vi "Tetra_BOUNCE_Setup.vi"() -> (0 "error out":errorcluster, 2 "Status":string="\rSetting up the Power Supplies...\rPower Supplies ON!\rMeasuring DC Power Supply Current(Pre-Boot)\rInitial DC = 0.144814  Amps")   [LabVIEW 2018]
uses:
  <vilib>/Utility/error.llb/DialogType.ctl
  Initialize References/Sequence Globals.vi
  Infrastructure/Test Parameter Globals_1.0.0.vi
  Tetra_Globals.vi
  Initialize References/Station References Global.vi
  Infrastructure/Test Result File Name Global.vi
  <vilib>/Utility/file.llb/Read Delimited Spreadsheet (string).vi
  <vilib>/Utility/file.llb/Write Delimited Spreadsheet (string).vi
panel:
  in  "Controls":T1={"ReadADC"=TRUE, "StartTest"=TRUE, "ResetRFSM"=TRUE, "FtServer"=TRUE, "CalVCO(t)"=TRUE, "Ping(t)"=TRUE, "CmdWindowHide(T)"=FALSE, "OpenNewFt(T)"=TRUE, "UseCmdFile(T)"=FALSE, "#of Retries"=5}
  out "COM PORT":string="COM6"
  out "bad usb connection?(t)":bool
  out "capt_dir":string="#CaptureFileDirectory: 'C:\\RageATE Results\\WAM-C_BOUNCE\\11_28_2022\\WAM-C_BOUNCE_SN_WAM-000102_ 2239_112822-151618_IqCaptureFiles.zip'"
  out "Pmic_FwRev":string
  out "snic":string="#Family: 0x2D\n#Serial: 0x000036092740\r\n"
  out "rev":string="rdiv\r\n0)  sw3p6:   195 mA  3616 mV\r\n1)  sw5p5:    89 mA  5472 mV\r\n2) sw2p8a:   315 mA  2784 mV\r\n3) sw2p8b:   349 mA  2768 mV\r\n4)  sw2p4:  1458 mA  2288 mV\r\n5)  sw1p4:  1047 mA  1304 mV\r\n>"
  out "Tab Control":enum32{"Page 1", "Page 2", "Page 3", "Page 4"}(tab)
  in  "CheckInputClock(T)":bool=TRUE
  in  "Setup Chip (T)":bool=TRUE
  in  "Setup Power Supply (T)":bool=TRUE
  in  "Kill Teraterm":bool=TRUE
  in  "Setup Gantry(t)":bool=TRUE
  out "FPGA_Booted":bool
  out "Ping_Success":bool
  out "Success":bool
  out "AminitOK?(t)":bool=TRUE
  out "Capt_RxIQ_Data(t)":bool=TRUE
  in  "RunFtVco/Ping(t)":bool=TRUE
  out "PyScript(path)":path=path "C:/RageATE/Automated Tests/Tetra WAM/Utilities/VerifySiTime.py"
  out "CMD":string
  out "AppSupportPath":path
  out "IsRuntime?":bool
  out "gui_path":path
  out "ft_path":path
  out "Use PS1-1":bool=TRUE
  out "Temp(t)":bool
  out "Text":refnum<vi>
  out "PS1-1(V)":dbl=18.75
  out "PS1-1(A)":dbl=1.0
  out "Temp Soak(min)":dbl caption="Delay Time (s)"
  out "-dynamic (t)":bool
  out "RunAM_Init(T)":bool
  out "RundynamicMode_Init(T)":bool
  out "PllSuccess?(T)":bool
  out "git log":string="#Gitlog Commit: bb6f7468ffd055d506c281d33be7af8cc293d965   Ver: 1.0.28\n#Gitlog Author: Rick-Rage <74794943+Rick-Rage@users.noreply.github.com>\n#Gitlog Date:   Wed Nov 23 09:45:19 2022 -0500\n#Gitlog ComputerName: HAMPTON"
  out "TEMP":dbl=25.0
  in  "error in (no error)":errorcluster
  # "CLOCK TEST FILES"
types:
  T1 = cluster{"ReadADC":bool, "StartTest":bool, "ResetRFSM":bool, "FtServer":bool, "CalVCO(t)":bool, "Ping(t)":bool, "CmdWindowHide(T)":bool, "OpenNewFt(T)":bool, "UseCmdFile(T)":bool, "#of Retries":i32}
  T2 = typedef "DialogType.ctl" = u16
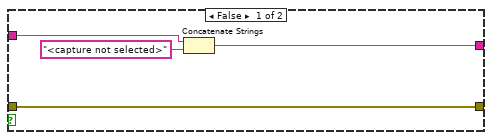
[diagram p3: hidden frame]
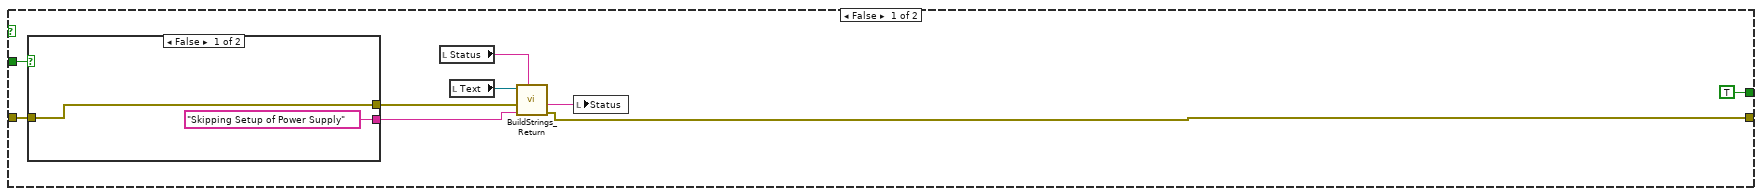
[diagram p5: hidden frame]
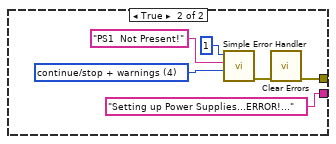
[diagram p6: hidden frame]
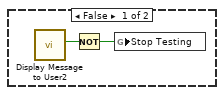
[diagram p8: hidden frame]
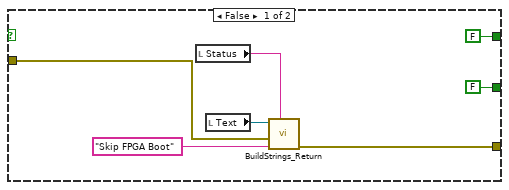
[diagram p10: hidden frame]
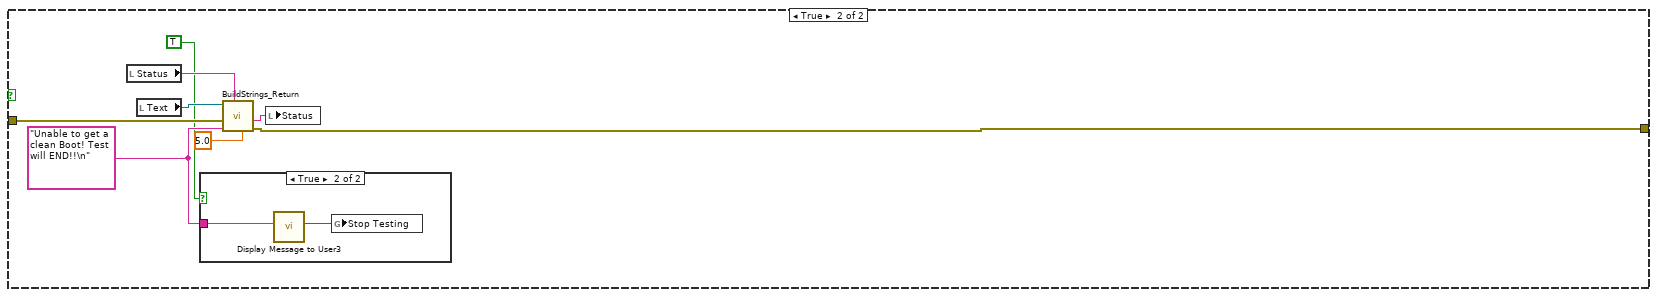
[diagram p11: hidden frame]
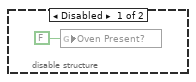
[diagram p13: hidden frame]
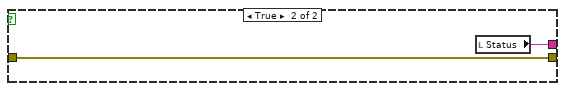
[diagram p14: hidden frame]
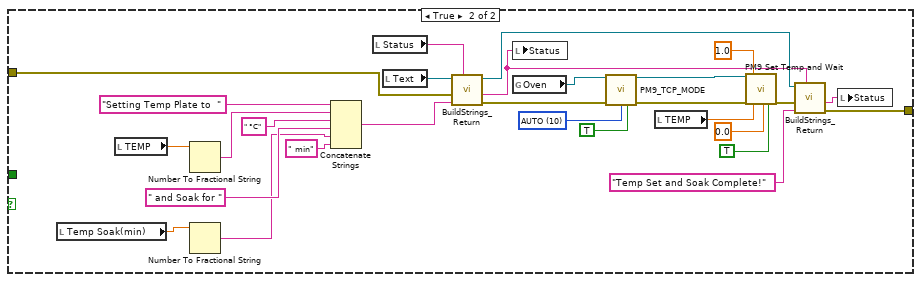
[diagram p15: hidden frame]
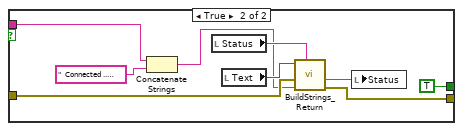
[diagram p17: hidden frame]
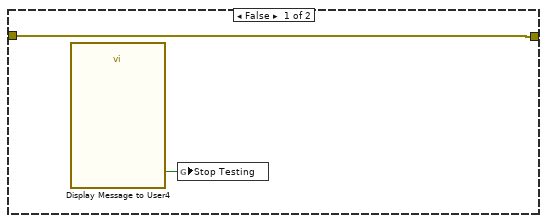
[diagram p19: hidden frame]
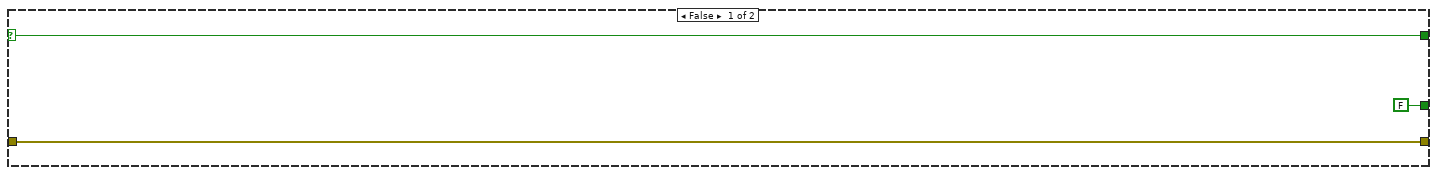
[diagram p20: hidden frame]
diagram:
  n1 = flat-sequence {
    tunnel: [w38] -> w15
    tunnel: w15 -> [w57]
    tunnel: [w56] -> w14
    tunnel: [w55] -> w13
    tunnel: [w53] -> w6
    tunnel: [w71] -> w7
    tunnel: w14 -> [w78]
    tunnel: w13 -> [w77]
    tunnel: w6 -> [w71]
    tunnel: [w81] -> w12
    tunnel: w7 -> [w80]
    tunnel: w12 -> [w103]
    tunnel: [w102] -> w11
    tunnel: [w113] -> w9
    tunnel: w11 -> [w112]
    tunnel: [w111] -> w1
    tunnel: w9 -> [w182]
    tunnel: [w181] -> w4
    tunnel: w1 -> [w180]
    tunnel: [w242] -> w5
    tunnel: w4 -> [w241]
    tunnel: [w293] -> w8
    tunnel: w5 -> [w294]
    tunnel: [w338] -> w3
    tunnel: w8 -> [w337]
    tunnel: w3 -> [w425]
    tunnel: [w424] -> w2
    tunnel: [w473] -> w10
    tunnel: w2 -> [w484]
    frame #0 {
      w16 = FALSE ("FPGA_Booted")
      # "Kill TeraTerm"
      n2 = flat-sequence {
        frame #0 {
          # "Clock Test References"
          n3 = global read "Sequence Globals.vi" "DevSupportPath"() -> (w43:path)
          n4 = global read "Sequence Globals.vi" "AppSupportPath"() -> (w45:path)
          "AppSupportPath" <- w45
          n5 = Strip Path(path=w43) -> (stripped path=w42:path)  [unwired: 1 out]
          n6 = global read "Sequence Globals.vi" "IsRuntime?"() -> (w46:bool)
          "IsRuntime?" <- w46
          n7 = Build Path(base path=w42, name or relative path=path "Utilities/VerifySiTime.py" ("PyScript(path)")) -> (appended path=w40:path)
          n8 = Select(t=w45, s=w46, f=w40) -> (s? t:f=w44:path)
          "PyScript(path)" <- w44
          n9 = local write "PyScript(path)"(w44) -> ()
        }
      }
      n10 = global read "Sequence Globals.vi" "DevSupportPath"() -> (w28:path)
      n11 = global read "Sequence Globals.vi" "DevSupportPath"() -> (w18:path)
      n12 = global read "Sequence Globals.vi" "RageATE_Gitlog"() -> (→"git log":string)
      n13 = local write "AminitOK?(t)"(w16) -> ()
      n14 = global read "Sequence Globals.vi" "AppSupportPath 3"() -> (w23:path)
      n15 = global read "Sequence Globals.vi" "AppSupportPath 3"() -> (w22:path)
      n16 = global read "Sequence Globals.vi" "IsRuntime?"() -> (w24:bool)
      n17 = global read "Sequence Globals.vi" "IsRuntime?"() -> (w21:bool)
      n18 = local write "Setup Gantry(t)"("Setup Gantry(t)") -> ()
      n19 = local write "Setup Chip (T)"("Setup Chip (T)") -> ()
      n20 = Build Path(base path=w28, name or relative path=path "TetraLabGUI" ("PyScript(path)")) -> (appended path=w26:path)
      n21 = Build Path(base path=w18, name or relative path=path "FieldTestApp" ("PyScript(path)")) -> (appended path=w20:path)
      n22 = local write "Setup Power Supply (T)"("Setup Power Supply (T)") -> ()
      n23 = Select(t=w23, s=w24, f=w26) -> (s? t:f=→"gui_path":path)
      n24 = Select(t=w22, s=w21, f=w20) -> (s? t:f=→"ft_path":path)
      n25 = case shown="True" "Kill Teraterm" {
        tunnel: "error in (no error)" -> [w47 w49]
        tunnel: [w47 w48] -> w38
        tunnel: "taskkill /f /im ttermpro.exe" ("command line") -> [_ w51]
        frame False {
        }
        frame True {
          n26 = call <vilib>:"Clear Errors.vi"("error in (no error)"=w49) -> ("error out"=w50:errorcluster)  [unwired: 5 in, 1 out]
          n27 = call <vilib>:"System Exec.vi"("error in (no error)"=w50, "command line"=w51) -> ("error out"=w52:errorcluster)  [unwired: 6 in, 3 out]
          n28 = call "Time Delay2"("error in (no error)"=w52) -> ("error out"=w48:errorcluster)  [unwired: 10 in]
        }
      }
      "Success" <- FALSE ("Success")
      "Status" <- ""
      "Tab Control" <- enum32{"Page 1", "Page 2", "Page 3", "Page 4"}."Page 1" ("Tab Control")
      "RundynamicMode_Init(T)" <- w16
      "RunAM_Init(T)" <- w16
      "-dynamic (t)" <- w16
    }
    frame #1 {
      # "0\t0\tCOMPORT\tname\n1\t0\tPS1-1 V;I\tVolt : Amp\n2\t0\tCycle_Power\tBool\n3\t0\tAverages\tnum\n4\t0\tCreate_iq_File\tbool\n5\t0\tTemp_Soak\tsec\n6\t0\tCMD\tcommand line\n7\t0\tUse_Gantry\tBool"
      n29 = property on="Status" class="Str"(error in=w57) -> (error out=w53:errorcluster, "Text"=→"Text":refnum<vi>)  [unwired: 1 in, 1 out]
      n30 = global read "Test Parameter Globals_1.0.0.vi" "Input Constants Out"() -> (w56:string[])
      n31 = global read "Test Parameter Globals_1.0.0.vi" "Test Parameters"() -> (w55:string[][])
    }
    frame #2 {
      w64 = 0 ("index (row)")
      n32 = Index Array(array=w78) -> (element #1=w63:string, element #2=w58:string, element #5=w62:string, element #6=w61:string, element #7=→"CMD":string, element #8=w59:string)  [unwired: 8 in, 2 out]
      n33 = Index Array(array=w77, index (row)=w64, index (col)=w64) -> (element=w65:string)
      n34 = global read "Tetra_Globals.vi" "comport"() -> (w67:refnum<visa-resource-name>)
      n35 = Empty String/Path?(string/path=w63) -> (empty?=w69:bool)
      n36 = call "TempControlWithBool.vi"("INPUT"=w65) -> ("out"=→"TEMP":dbl, "Valid(t)"=w75:bool)  [unwired: 6 in, 1 out]
      "Temp(t)" <- w75
      n37 = call "StringToNumberControlWithBool(x2).vi"("string"=w58) -> ("Num(2)"=→"PS1-1(A)":dbl, "Num"=→"PS1-1(V)":dbl, "NOT_0?"=→"Use PS1-1":bool)  [unwired: 4 in, 4 out]
      n38 = call "StringToNumberControlWithBool.vi"("String In"=w62) -> ("NOT = 0"=→"Capt_RxIQ_Data(t)":bool)  [unwired: 7 in, 1 out]
      n39 = call "StringToNumberControlWithBool.vi"("String In"=w61) -> ("Number Out"=→"Temp Soak(min)":dbl)  [unwired: 7 in, 1 out]
      n40 = call "StringToNumberControlWithBool.vi"("String In"=w59) -> ("NOT = 0"=w66:bool)  [unwired: 7 in, 1 out]
      n41 = Select(t=w67, s=w69, f=w58) -> (s? t:f=→"COM PORT":refnum<visa-resource-name>)
      n42 = global write "Station References Global.vi" "Oven Present?"(w75) -> ()
      n43 = local write "Setup Gantry(t)"(w66) -> ()
    }
    frame #3 {
      n44 = flat-sequence {
        tunnel: w80 -> [w86]
        tunnel: [w85] -> w81
        frame #0 {
          n45 = local read "Capt_RxIQ_Data(t)"() -> (w82:bool)
          n46 = case shown="True" w82 {
            tunnel: [w87 w93] -> w84
            tunnel: w86 -> [w90 w97]
            tunnel: [w90 w96] -> w85
            tunnel: "#CaptureFileDirectory: " ("string") -> [w89 w95]
            frame False {
              n47 = Concatenate Strings(w89, "<capture not selected>" ("string")) -> (w87:string)
            }
            frame True {
              w94 = "'" ("string")
              # "For Header"
              n48 = global read "Test Result File Name Global.vi" "Test Results File Name"() -> (w101:path)
              n49 = Path To String(path=w101) -> (string=w100:string)
              n50 = Search and Replace String(input string=w100, search string=".csv", replace string="_Iq.csv" ("name or relative path"), error in=w97) -> (result string=w91:string, error out=w96:errorcluster)  [unwired: 4 in, 2 out]
              n51 = String To Path(string=w91) -> (path=w92:path)
              n52 = Concatenate Strings(w95, w94, w91, w94) -> (w93:string)
              n53 = global write "Tetra_Globals.vi" "TraceFilePath"(w92) -> ()
            }
          }
          "capt_dir" <- w84
        }
      }
    }
    frame #4 {
      n54 = global read "Station References Global.vi" "RF Switch Present?"() -> (w104:bool)
      n55 = case shown="True" w104 {
        tunnel: w103 -> [w105 w109]
        tunnel: [w105 w108] -> w102
        frame False {
        }
        frame True {
          n56 = global read "Station References Global.vi" "RF Switch"() -> (w110:refnum<visa-resource-name>)
          n57 = call "RfSwitch_WAM_ATE.vi"("VISA_IN"=w110, "error in"=w109, "Source"=enum16{"RFSM", "PNA"}."RFSM", "T/R"=enum16{"TX", "RX"}."RX") -> ("error out"=w108:errorcluster)  [unwired: 10 in, 1 out]
        }
      }
    }
    frame #5 {
      n58 = local read "Setup Power Supply (T)"() -> (w114:bool)
      n59 = global read "Station References Global.vi" "PS1 Present?"() -> (w116:bool)
      n60 = And(x=w116, y=w114) -> (x .and. y?=w115:bool)
      n61 = case shown="True" w115 {
        tunnel: [w119 w140] -> w113
        tunnel: w114 -> [w125 _]
        tunnel: w112 -> [w118 w139]
        tunnel: [TRUE w134] -> w111
        frame False {
          n62 = case shown="False" w125 {
            tunnel: [w126 w129] -> w120
            tunnel: ["Skipping Setup of Power Supply" "Setting up Power Supplies...ERROR!..."] -> w121
            tunnel: w118 -> [w126 _]
            frame False {
            }
            frame True {
              w131 = T2 4 items=["no dialog", "OK message", "continue or stop message", "OK message + warnings", "continue/stop + warnings"] ("type of dialog (OK msg:1)")
              n63 = call <vilib>:"Simple Error Handler.vi"("error code (no error:0)"=1, "error source (\" \")"="PS1  Not Present!" ("error source (\" \")"), "type of dialog (OK msg:1)"=w131) -> ("error out"=w130:errorcluster)  [unwired: 2 in, 4 out]
              n64 = call <vilib>:"Clear Errors.vi"("error in (no error)"=w130) -> ("error out"=w129:errorcluster)  [unwired: 5 in, 1 out]
            }
          }
          n65 = local read "Status"() -> (w122:string)
          n66 = local read "Text"() -> (w124:refnum<vi>)
          n67 = call "BuildStrings_Return.vi"("Input String"=w122, "New String"=w121, "error in (no error)"=w120, "reference"=w124) -> ("error out"=w119:errorcluster, "concatenated string"=w123:string)  [unwired: 5 in, 1 out]
          n68 = local write "Status"(w123) -> ()
        }
        frame True {
          n69 = control-ref of="Text"() -> ()  [unwired: 1 out]
          n70 = for {
            N: 2 -> [w145]
            shift-right: [w150] -> w140
            shift-left: w139 -> [w146]
            tunnel: [w142] -> w137
            tunnel: [w141] -> w136
            i -> [w144]
            stop <- w141 stop-if-true
            w148 = TRUE ("Open Ser(t)")
            n71 = Increment(x=w144) -> (x+1=w143:i32)
            n72 = Equal?(x=w145, y=w143) -> (x = y?=w142:bool)
            n73 = local read "Status"() -> (w159:string)
            n74 = local read "Text"() -> (w158:refnum<vi>)
            n75 = call "BuildStrings_Return.vi"("Input String"=w159, "New String"="Setting up the Power Supplies...", "error in (no error)"=w146, "reference"=w158) -> ("error out"=w160:errorcluster, "concatenated string"=w157:string)  [unwired: 5 in, 1 out]
            n76 = local write "Status"(w157) -> ()
            n77 = stacked-sequence {
              tunnel: w160 -> [w179]
              tunnel: [w178] -> w154
              tunnel: [w165] -> _
              tunnel: [w164] -> _
              frame #0 {
                w167 = "PS1" ("SEL_PS")
                # "Conf I/V lim"
                n78 = local read "Text"() -> (w170:refnum<vi>)
                n79 = local read "PS1-1(A)"() -> (w176:dbl)
                n80 = local read "PS1-1(V)"() -> (w175:dbl)
                n81 = property class="Txt"(reference=w170, error in=w179, "Scroll Position"=i16 -1) -> (error out=w168:errorcluster)  [unwired: 1 out]
                n82 = global read "Station References Global.vi" "PS1"() -> (w177:refnum<visa-resource-name>)
                n83 = Build Array(w176, 1.0 ("element")) -> (w165:dbl[])
                n84 = Build Array(w175, 5.0 ("element")) -> (w164:dbl[])
                n85 = call "PS_SETUP_V-I-EN.vi"("VISA resource name"=w177, "SEL_PS"=w167, "error in (no error)"=w168, "Use Channel"=bool[] [FALSE, FALSE, FALSE, FALSE], "Current Lim"=w165, "Voltage Set"=w164) -> ("VISA resource name out"=w171:refnum<visa-resource-name>, "error out"=w173:errorcluster)  [unwired: 8 in]
                n86 = call "Time Delay5"("error in (no error)"=w173) -> ("error out"=w166:errorcluster)  [unwired: 10 in]
                n87 = call "PS_SETUP_V-I-EN.vi"("VISA resource name"=w171, "SEL_PS"=w167, "error in (no error)"=w166, "Use Channel"=bool[] [TRUE, FALSE, FALSE, FALSE], "Current Lim"=w165, "Voltage Set"=w164) -> ("error out"=w178:errorcluster)  [unwired: 8 in, 1 out]
              }
            }
            n88 = local read "Text"() -> (w156:refnum<vi>)
            n89 = local read "COM PORT"() -> (w149:string)
            n90 = call "BuildStrings_Return.vi"("seconds to wait"=5.0, "Input String"=w157, "New String"="Power Supplies ON!", "error in (no error)"=w154, "reference"=w156) -> ("error out"=w151:errorcluster, "concatenated string"=w153:string)  [unwired: 4 in, 1 out]
            n91 = local write "Status"(w153) -> ()
            n92 = call "Tetra Serial.vi"("COMPORT"=w149, "ClearErrorIn(t)"=TRUE, "error in (no error)"=w151, "Open Ser(t)"=w148, "Close Ser(t)"=w148) -> ("Success"=w141:bool, "error out"=w150:errorcluster)  [unwired: 6 in, 3 out]
          }
          n93 = Not(x=w136) -> (.not. x?=w135:bool)
          n94 = And(x=w137, y=w135) -> (x .and. y?=w134:bool)
          "bad usb connection?(t)" <- w134
        }
      }
    }
    frame #6 {
      n95 = case shown="False" w180 {
        tunnel: w182 -> [w184 w234]
        tunnel: [w183 w230] -> w181
        frame False {
          n96 = flat-sequence {
            tunnel: w184 -> [w192]
            tunnel: [w187] -> w183
            frame #0 {
              n97 = local read "Setup Chip (T)"() -> (w193:bool)
              n98 = case shown="True" w193 {
                selector: w193 -> [_ w217]
                tunnel: [FALSE ("Success") w229] -> w188
                tunnel: [w210 w216] -> w191
                tunnel: w192 -> [w211 w220]
                tunnel: [FALSE w217] -> w189
                frame False {
                  n99 = local read "Status"() -> (w212:string)
                  n100 = local read "Text"() -> (w213:refnum<vi>)
                  n101 = call "BuildStrings_Return.vi"("Input String"=w212, "New String"="Skip FPGA Boot", "error in (no error)"=w211, "reference"=w213) -> ("error out"=w210:errorcluster)  [unwired: 5 in, 2 out]
                }
                frame True {
                  n102 = local read "Status"() -> (w224:string)
                  n103 = local read "Text"() -> (w223:refnum<vi>)
                  n104 = call "BuildStrings_Return.vi"("seconds to wait"=0.0, "Input String"=w224, "New String"="Booting up FPGA...\nTakes up to 10sec..." ("Delay text ..."), "error in (no error)"=w220, "reference"=w223) -> ("error out"=w219:errorcluster, "concatenated string"=w218:string)  [unwired: 4 in, 1 out]
                  n105 = local read "COM PORT"() -> (w226:string)
                  n106 = local write "Status"(w218) -> ()
                  n107 = call "Tetra Serial.vi"("COMPORT"=w226, "error in (no error)"=w219, "Command"="", "Open Ser(t)"=TRUE, "Close Ser(t)"=FALSE) -> ("Success"=w229:bool, "error out"=w216:errorcluster)  [unwired: 6 in, 3 out]
                }
              }
              n108 = And(x=w188, y=w189) -> (x .and. y?=w190:bool)
              n109 = local write "FPGA_Booted"(w188) -> ()
              n110 = case shown="True" w190 {
                tunnel: w191 -> [w202 w207]
                tunnel: [w202 w203] -> w186
                frame False {
                }
                frame True {
                  n111 = local read "Status"() -> (w206:string)
                  n112 = local read "Text"() -> (w208:refnum<vi>)
                  n113 = call "BuildStrings_Return.vi"("Input String"=w206, "New String"="FPGA Success!!", "error in (no error)"=w207, "reference"=w208) -> ("error out"=w203:errorcluster, "concatenated string"=w204:string)  [unwired: 5 in, 1 out]
                  n114 = local write "Status"(w204) -> ()
                }
              }
              n115 = local read "CheckInputClock(T)"() -> (w185:bool)
              n116 = case shown="True" w185 {
                tunnel: [w194 w199] -> w187
                tunnel: w186 -> [w194 w198]
                frame False {
                }
                frame True {
                  w195 = u16 0 items=["EXT CLK", "INT CLK"] ("CLK_USAGE")
                  n117 = local read "COM PORT"() -> (w196:string)
                  n118 = call "InputClk_Status.vi"("COMPORT"=w196, "error in (no error)"=w198, "CLK_USAGE"=w195) -> ("PllSuccess?(T)"=w197:bool, "error out"=w199:errorcluster)  [unwired: 11 in]
                  "PllSuccess?(T)" <- w197
                  n119 = case shown="True" w197 {
                    frame False {
                      n120 = call "Display Message to User2"() -> ("OK"=w201:bool)  [unwired: 10 in, 1 out]
                      n121 = Not(x=w201) -> (.not. x?=w200:bool)
                      n122 = global write "Sequence Globals.vi" "Stop Testing"(w200) -> ()
                    }
                    frame True {
                    }
                  }
                }
              }
            }
          }
        }
        frame True {
          w232 = "Unable to get a clean Boot! Test will END!!\n" ("New String")
          n123 = local read "Status"() -> (w233:string)
          n124 = local read "Text"() -> (w235:refnum<vi>)
          n125 = case shown="True" TRUE {
            tunnel: w232 -> [_ w239]
            frame False {
            }
            frame True {
              n126 = call "Display Message to User3"("Message"=w239) -> ("OK"=w238:bool)  [unwired: 9 in, 1 out]
              n127 = global write "Sequence Globals.vi" "Stop Testing"(w238) -> ()
            }
          }
          n128 = call "BuildStrings_Return.vi"("seconds to wait"=5.0, "Input String"=w233, "New String"=w232, "error in (no error)"=w234, "reference"=w235) -> ("error out"=w230:errorcluster, "concatenated string"=w236:string)  [unwired: 4 in, 1 out]
          n129 = local write "Status"(w236) -> ()
        }
      }
    }
    frame #7 {
      n130 = global read "Sequence Globals.vi" "Stop Testing"() -> (w240:bool)
      n131 = case shown="False" w240 {
        tunnel: [w244 w291] -> w242
        tunnel: w241 -> [w243 w291]
        frame False {
          n132 = global read "Station References Global.vi" "Oven Present?"() -> (w245:bool)
          n133 = local read "Temp(t)"() -> (w246:bool)
          n134 = And(x=w246, y=w245) -> (x .and. y?=w247:bool)
          n135 = case shown="False" w247 {
            tunnel: w246 -> [w253 _]
            tunnel: [w251 w273] -> w244
            tunnel: w243 -> [w248 w286]
            frame False {
              n136 = disable-structure shown="Enabled" {
                frame Disabled {
                  n137 = global write "Station References Global.vi" "Oven Present?"(FALSE ("Oven Present?")) -> ()
                }
                frame Enabled {
                }
              }
              n138 = call "Display Message to User"("error in (no error)"=w248, "Enable"=w253) -> ("error out"=w250:errorcluster, "Cancel"=w252:bool)  [unwired: 8 in]
              n139 = Stop(stop? (T)=w252) -> ()
              n140 = case shown="False" w252 {
                tunnel: [w259 w261] -> w249
                tunnel: [w258 w262] -> w251
                tunnel: w250 -> [w257 w262]
                frame False {
                  n141 = local read "Status"() -> (w255:string)
                  n142 = local read "Text"() -> (w256:refnum<vi>)
                  n143 = call "BuildStrings_Return.vi"("Input String"=w255, "New String"="Skipping Setting Up Temperature...", "error in (no error)"=w257, "reference"=w256) -> ("error out"=w258:errorcluster, "concatenated string"=w259:string)  [unwired: 5 in, 1 out]
                }
                frame True {
                  n144 = local read "Status"() -> (w261:string)
                }
              }
              n145 = local write "Status"(w249) -> ()
            }
            frame True {
              w281 = u16 10 items=["READ ONLY"=0, "AUTO"=10, "OFF"=62, "MAN"=54] ("MODE")
              n146 = local read "Temp Soak(min)"() -> (w269:dbl)
              n147 = local read "TEMP"() -> (w276:dbl)
              n148 = Number To Fractional String(number=w276) -> (F-format string=w275:string)  [unwired: 3 in]
              n149 = Number To Fractional String(number=w269) -> (F-format string=w267:string)  [unwired: 3 in]
              n150 = Concatenate Strings("Setting Temp Plate to  ", w275, " °C" ("string"), " and Soak for " ("string"), w267, " min" ("string")) -> (w277:string)
              n151 = local read "Status"() -> (w278:string)
              n152 = local read "Text"() -> (w279:refnum<vi>)
              n153 = call "BuildStrings_Return.vi"("Input String"=w278, "New String"=w277, "error in (no error)"=w286, "reference"=w279) -> ("error out"=w283:errorcluster, "concatenated string"=w264:string, "reference out"=w271:refnum<vi>)  [unwired: 5 in]
              n154 = local write "Status"(w264) -> ()
              n155 = global read "Station References Global.vi" "Oven"() -> (w284:refnum<visa-resource-name>)
              n156 = call "PM9_TCP_MODE.vi"("VISA"=w284, "error in (no error)"=w283, "MODE"=w281, "Close tcp(t)"=TRUE) -> ("visa out"=w280:refnum<visa-resource-name>, "error out"=w285:errorcluster)  [unwired: 8 in, 2 out]
              n157 = local read "TEMP"() -> (w289:dbl)
              n158 = call "PM9 Set Temp and Wait.vi"("VISA"=w280, "Error In"=w285, "Accuracy +/-"=1.0, "Set Point"=w289, "Min (-1 for cont.)"=0.0, "close session(t)"=TRUE) -> ("error out"=w272:errorcluster)  [unwired: 10 in, 3 out]
              n159 = call "BuildStrings_Return.vi"("Input String"=w264, "New String"="Temp Set and Soak Complete!", "error in (no error)"=w272, "reference"=w271) -> ("error out"=w273:errorcluster, "concatenated string"=w270:string)  [unwired: 5 in, 1 out]
              n160 = local write "Status"(w270) -> ()
            }
          }
        }
        frame True {
        }
      }
    }
    frame #8 {
      n161 = global read "Sequence Globals.vi" "Stop Testing"() -> (w292:bool)
      n162 = case shown="False" w292 {
        tunnel: w294 -> [w300 w335]
        tunnel: [w299 w335] -> w293
        frame False {
          n163 = for {
            N: 2 -> [_]
            shift-right: [w306] -> w299
            shift-left: w300 -> [w310]
            tunnel: [w303] -> w298
            stop <- w303 stop-if-true
            n164 = local read "Status"() -> (w311:string)
            n165 = local read "Text"() -> (w313:refnum<vi>)
            n166 = call "BuildStrings_Return.vi"("seconds to wait"=1.0, "Input String"=w311, "New String"="Checking IP Address: 169.254.70.191, for Fast RxData", "error in (no error)"=w310, "reference"=w313) -> ("error out"=w307:errorcluster, "concatenated string"=w309:string)  [unwired: 4 in, 1 out]
            n167 = local write "Status"(w309) -> ()
            n168 = call "PingCmdLine.vi"("error in (no error)"=w307, "IP Address"="169.254.70.191" ("IP_ADDR")) -> ("error out"=w308:errorcluster, "Match?(t)"=w301:bool, "Ip_out"=w302:string)  [unwired: 7 in]
            n169 = case shown="False" w301 {
              tunnel: w308 -> [w319 w331]
              tunnel: [w317 w330] -> w306
              tunnel: [w316 TRUE] -> w303
              tunnel: w302 -> [w314 w326]
              frame False {
                n170 = Concatenate Strings("Failed to Connect to " ("New String"), w314, "Check Address and Connections" ("string")) -> (w322:string)
                n171 = local read "Status"() -> (w324:string)
                n172 = local read "Text"() -> (w323:refnum<vi>)
                n173 = call "BuildStrings_Return.vi"("Input String"=w324, "New String"=w322, "error in (no error)"=w319, "reference"=w323) -> ("error out"=w318:errorcluster, "concatenated string"=w325:string)  [unwired: 5 in, 1 out]
                n174 = local write "Status"(w325) -> ()
                n175 = call "Prompt User for Input2"("Enable"=TRUE, "error in (no error)"=w318) -> ("OK"=w316:bool, "error out"=w317:errorcluster)  [unwired: 16 in]
              }
              frame True {
                n176 = Concatenate Strings(w326, "  Connected ..Success!!" ("New String")) -> (w329:string)
                n177 = local read "Status"() -> (w333:string)
                n178 = local read "Text"() -> (w332:refnum<vi>)
                n179 = call "BuildStrings_Return.vi"("Input String"=w333, "New String"=w329, "error in (no error)"=w331, "reference"=w332) -> ("error out"=w330:errorcluster, "concatenated string"=w334:string)  [unwired: 5 in, 1 out]
                n180 = local write "Status"(w334) -> ()
              }
            }
            n181 = local write "Ping_Success"(w303) -> ()
          }
          n182 = local read "FPGA_Booted"() -> (w296:bool)
          n183 = And(x=w296, y=w298) -> (x .and. y?=w297:bool)
          n184 = local write "Success"(w297) -> ()
        }
        frame True {
        }
      }
    }
    frame #9 {
      n185 = global read "Sequence Globals.vi" "Stop Testing"() -> (w336:bool)
      n186 = case shown="False" w336 {
        tunnel: [w347 w422] -> w338
        tunnel: w337 -> [w340 w422]
        frame False {
          n187 = local read "Setup Chip (T)"() -> (w342:bool)
          n188 = local read "Success"() -> (w341:bool)
          n189 = And(x=w342, y=w341) -> (x .and. y?=w343:bool)
          n190 = case shown="True" w343 {
            selector: w343 -> [w374 w403]
            tunnel: w340 -> [w375 w382]
            tunnel: [w375 w378] -> w345
            tunnel: [w374 w403] -> w346
            tunnel: [FALSE ("OK?(t)") w376] -> w339
            frame False {
            }
            frame True {
              n191 = local read "CMD"() -> (w391:string)
              n192 = Empty String/Path?(string/path=w391) -> (empty?=w392:bool)
              n193 = case shown="False" w392 {
                tunnel: [w419 ""] -> w381
                tunnel: w391 -> [w418 _]
                frame False {
                  n194 = Concatenate Strings(";" ("string"), w418) -> (w419:string)
                }
                frame True {
                }
              }
              n195 = local read "COM PORT"() -> (w383:string)
              n196 = call "SerRW-Array.vi"("COMPORT"=w383, "error in (no error)"=w382, "Command ( ; seperation)"=w381, "Open Serial"=FALSE ("Open/Close Serial")) -> ("comport"=w395:refnum<visa-resource-name>, "error out"=w394:errorcluster)  [unwired: 5 in, 5 out]
              n197 = global read "Tetra_Globals.vi" "BarCodeESN"() -> (w384:string)
              n198 = call "Tetra_Rev.vi"("COMPORT"=w395, "error in (no error)"=w394) -> ("rev"=→"rev":string, "comport"=w401:refnum<visa-resource-name>, "error out"=w400:errorcluster)  [unwired: 9 in, 2 out]
              n199 = call "Tetra_ReadESN.vi"("COMPORT"=w401, "BC_Esn"=w384, "error in (no error)"=w400) -> ("read"=→"snic":string, "comport"=w387:refnum<visa-resource-name>, "esn"=w398:string, "error out"=w389:errorcluster)  [unwired: 8 in, 1 out]
              n200 = global write "Tetra_Globals.vi" "ESN"(w398) -> ()
              n201 = call "ESNLookup.vi"("ESN"=w398, "error in"=w389) -> ("error out"=w388:errorcluster)  [unwired: 7 in, 2 out]
              n202 = call "UCD_Device-Info.vi"("COMPORT"=w387, "error in (no error)"=w388) -> ("Pmic_FwRev"=→"Pmic_FwRev":string, "comport"=w377:refnum<visa-resource-name>, "error out"=w386:errorcluster)  [unwired: 10 in, 1 out]
              n203 = local read "Status"() -> (w396:string)
              n204 = local read "Text"() -> (w397:refnum<vi>)
              n205 = call "BuildStrings_Return.vi"("Input String"=w396, "error in (no error)"=w386, "reference"=w397) -> ("error out"=w380:errorcluster, "concatenated string"=w390:string)  [unwired: 6 in, 1 out]
              n206 = local write "Status"(w390) -> ()
              n207 = case shown="True" "RunFtVco/Ping(t)" {
                tunnel: w380 -> [w405 w417]
                tunnel: [w405 w416] -> w378
                tunnel: w377 -> [_ w414]
                tunnel: [TRUE ("OK?(t)") w415] -> w376
                frame False {
                }
                frame True {
                  w407 = FALSE ("UseCmdFile(T)")
                  w408 = TRUE ("ReadADC")
                  n208 = Bundle By Name(cluster="Controls", "StartTest"=w408, "ResetRFSM"=w408, "FtServer"=w408, "OpenNewFt(T)"=w408, "CalVCO(t)"=w408, "Ping(t)"=w408, "CmdWindowHide(T)"=w408, "UseCmdFile(T)"=w407, "ReadADC"=w407, "#of Retries"=0) -> (w409:T1)
                  n209 = local read "gui_path"() -> (w413:path)
                  n210 = local read "ft_path"() -> (w412:path)
                  n211 = call "Bounce(LC).vi"("COMPORT"=w414, "Gui(path)"=w413, "Ft directory"=w412, "error in (no error)"=w417, "Controls"=w409, "Standalone vi(t)"=FALSE) -> ("PingOK?(t)"=w415:bool, "error out"=w416:errorcluster)  [unwired: 4 in, 4 out]
                  "AminitOK?(t)" <- w415
                }
              }
            }
          }
          n212 = And(x=w346, y=w339) -> (x .and. y?=w344:bool)
          n213 = case shown="True" w344 {
            tunnel: w345 -> [w349 w350]
            tunnel: [w349 w351] -> w347
            frame False {
              n214 = call "Display Message to User4"() -> ("END"=w348:bool)  [unwired: 10 in, 1 out]
              n215 = global write "Sequence Globals.vi" "Stop Testing"(w348) -> ()
            }
            frame True {
              n216 = flat-sequence {
                tunnel: [w366] -> w351
                tunnel: w350 -> [w357]
                frame #0 {
                  w353 = "\r\n"
                  n217 = local read "git log"() -> (w352:string)
                  n218 = global read "Test Parameter Globals_1.0.0.vi" "OperatorInfo"() -> (w364:string)
                  n219 = global read "Test Parameter Globals_1.0.0.vi" "BarCodeInfo"() -> (w363:string)
                  n220 = local read "Pmic_FwRev"() -> (w360:string)
                  n221 = global read "Test Result File Name Global.vi" "Test Results File Name"() -> (w355:path)
                  n222 = local read "capt_dir"() -> (w354:string)
                  n223 = local read "snic"() -> (w361:string)
                  n224 = call <vilib>:"Trim Whitespace.vi"("string"=w352) -> ("trimmed string"=w359:string)  [unwired: 1 in]
                  n225 = local read "rev"() -> (w362:string)
                  n226 = Concatenate Strings(w364, w353, w363, w362, w361, w360, w353, w359, w353, w354, w353) -> (w358:string)
                  n227 = call-poly <vilib>:"Read Delimited Spreadsheet.vi"("file path (dialog if empty)"=w355, "error in (no error)"=w357) -> ("new file path (Not A Path if cancelled)"=w371:path, "all rows"=w372:string[][], "error out"=w367:errorcluster)  [unwired: 8 in, 3 out]
                  n228 = Build Array(w358) -> (w356:string[])
                  n229 = Insert Into Array(array=w372, index (row)=0, new element=w356) -> (w369:string[][])  [unwired: 1 in]
                  n230 = call-poly <vilib>:"Write Delimited Spreadsheet.vi"("file path (dialog if empty)"=w371, "2D data"=w369, "append to file? (new file:F)"=FALSE, "error in (no error)"=w367, "delimiter (\\t)"="," ("delimiter (\\t)")) -> ("error out"=w366:errorcluster)  [unwired: 9 in, 1 out]
                }
              }
            }
          }
        }
        frame True {
        }
      }
    }
    frame #10 {
      n231 = global read "Sequence Globals.vi" "Stop Testing"() -> (w423:bool)
      n232 = case shown="False" w423 {
        tunnel: w425 -> [w427 w468]
        tunnel: [w426 w468] -> w424
        frame False {
          n233 = global read "Station References Global.vi" "Gantry Present?"() -> (w429:bool)
          n234 = local read "Setup Gantry(t)"() -> (w430:bool)
          n235 = And(x=w430, y=w429) -> (x .and. y?=w428:bool)
          n236 = case shown="True" w428 {
            tunnel: w427 -> [w431 w435]
            tunnel: [w431 w446] -> w426
            frame False {
            }
            frame True {
              w432 = u16 0 items=["HOME", "TX1", "TX2", "TX3", "TX4", "TX5", "TX6", "TX7", "TX8", "TX9", "TX10", "TX11", "TX12", "RX8", "RX7", "RX6", "RX5", "RX4", "RX3", "RX2", "RX1"] ("Antenna Select")
              w437 = u16 0 items=["Inches", "cm"] ("Zunits")
              n237 = global read "Station References Global.vi" "Gantry"() -> (w433:refnum<visa-resource-name>)
              n238 = for {
                N: 2 -> [_]
                tunnel: w433 -> [w456]
                shift-right: [w451] -> w436
                shift-left: w435 -> [w455]
                tunnel: [w448] -> _
                stop <- w449 stop-if-true
                w454 = TRUE ("Open Serial")
                n239 = call "WAM_ESS.vi"("VISA resource name"=w456, "error in (no error)"=w455, "Open Serial"=w454, "Test Running (T)"=w454, "Close Serial"=w454) -> ("Enabled(T-RO)"=w453:bool, "FH_NOT(T)"=w452:bool, "VISA resource name out"=w447:refnum<visa-resource-name>, "error out"=w450:errorcluster)  [unwired: 7 in]
                n240 = And(x=w453, y=w452) -> (x .and. y?=w449:bool)
                n241 = case shown="False" w449 {
                  tunnel: [w465 w467] -> w451
                  tunnel: w450 -> [w463 w467]
                  tunnel: [w460 w466] -> w448
                  tunnel: w447 -> [w459 w466]
                  frame False {
                    w457 = TRUE ("Close Serial")
                    w458 = u16 1 items=["Disable Driver", "Enable Driver", "Read Driver Status"] ("Driver-Func")
                    n242 = call "Prompt User for Input3"("error in (no error)"=w463) -> ("RESET"=w462:bool, "error out"=w464:errorcluster)  [unwired: 17 in]
                    n243 = Not(x=w462) -> (.not. x?=w461:bool)
                    n244 = Stop(stop? (T)=w461) -> ()
                    n245 = call "Gantry_Driver.vi"("VISA resource name"=w459, "error in (no error)"=w464, "Open Serial"=w457, "Driver-Func"=w458, "Close Serial"=w457) -> ("VISA resource name out"=w460:refnum<visa-resource-name>, "error out"=w465:errorcluster)  [unwired: 11 in, 2 out]
                  }
                  frame True {
                  }
                }
              }
              n246 = local read "Status"() -> (w444:string)
              n247 = local read "Text"() -> (w443:refnum<vi>)
              n248 = global read "Station References Global.vi" "Gantry"() -> (w439:refnum<visa-resource-name>)
              n249 = call "BuildStrings_Return.vi"("Input String"=w444, "New String"="Setting up Gantry", "error in (no error)"=w436, "reference"=w443) -> ("error out"=w441:errorcluster, "concatenated string"=w440:string)  [unwired: 5 in, 1 out]
              n250 = local write "Status"(w440) -> ()
              n251 = call "Gantry.vi"("COMPORT"=w439, "error in (no error)"=w441, "Antenna Select"=w432, "z ref"=21.0, "Write(reads antenna co-ords when off)"=TRUE, "Zunits"=w437) -> ("error out"=w446:errorcluster)  [unwired: 13 in]
            }
          }
        }
        frame True {
        }
      }
    }
    frame #11 {
      n252 = local read "bad usb connection?(t)"() -> (w472:bool)
      n253 = control-ref of="This VI"() -> (w483:refnum<vi>)
      n254 = property class="VI"(reference=w483) -> ("Path"=w481:path)  [unwired: 1 in, 2 out]
      n255 = Select(t="There was a problem setting up the DUT. Test Ended" ("New String"), s=w472, f="Setup Complete !!!" ("New String")) -> (s? t:f=w469:string)
      n256 = local read "Status"() -> (w486:string)
      n257 = local read "Text"() -> (w485:refnum<vi>)
      n258 = Path To String(path=w481) -> (string=w482:string)
      n259 = call "BuildStrings_Return.vi"("seconds to wait"=2.0, "Input String"=w486, "New String"=w469, "error in (no error)"=w484, "reference"=w485) -> ("error out"=w474:errorcluster, "concatenated string"=w476:string)  [unwired: 4 in, 1 out]
      n260 = Search and Replace String(input string=w482, search string=".vi", replace string=".txt" ("replace string (\"\")")) -> (result string=w477:string)  [unwired: 5 in, 3 out]
      n261 = local write "Status"(w476) -> ()
      n262 = String To Path(string=w477) -> (path=w478:path)
      n263 = Build Array(w476) -> (w475:string[])
      n264 = call-poly <vilib>:"Write Delimited Spreadsheet.vi"("file path (dialog if empty)"=w478, "1D data"=w475, "error in (no error)"=w474) -> ("error out"=w473:errorcluster)  [unwired: 11 in, 1 out]
    }
  }
  "error out" <- w10
